vi "manip_linearize.vi"(6 "Reset":bool, 7 "Parameters":T1={"Stimulus"={"Type"=enum."Off", "Phase"=0.0, "Amplitude"=[], "Injection point"=enum."Total pose", "Closed loop"=FALSE, "Offset"=[], "Tip -> world"=FALSE, "Frequency"=0.0, "Length"=0.0}, "Goal Filter A"={"Speedup max"=0.0, "Speedup thresh"=0.0, "Speedup nonlin"=0.0, "Filters"=[]}, "Mode controls"={"Hold"=FALSE, "Cancellation"=FALSE, "Goal filter"=FALSE, "Trigger"=FALSE}, "Manipulator type"=enum."Current piezo", "Manipulator calibration"={"Tool offsets"=[[0.0, 0.0, 36200.0]], "Tip light calibration"=[], "Handle light calibration"=[], "Base pivots"=[], "Output pivots"=[], "Length center"=0.0, "Workspace height"=[], "Workspace diameter"=[0.0, 0.0, 36200.0], "Linearization"=[[0.0, 0.0, 36200.0]], "Stack travel"=400.0, "Saturation pos"=375.0, "Inverse filters"=[]}, "Network"={"Remote Host"="", "Send Status"=FALSE, "Send Port"=0, "Recv Commands"=FALSE, "Recv Port"=0}, "Goal Filter B"={"Speedup max"=0.0, "Speedup thresh"=0.0, "Speedup nonlin"=0.0, "Filters"=[]}, "Cancellation"={"KP"={"XY"=0.0, "Rxy"=0.0, "Z"=0.0, "Rz"=0.0}, "KI"=0.0, "KD"={"XY"=0.0, "Rxy"=0.0, "Z"=0.0, "Rz"=0.0}, "Max vel"=20.0, "Max acc"=0.001, "Int error limit"=3.0, "RCM gain"=0.0, "Bypass"=FALSE, "Degraded gain"=0.0}, "Transition time"=0.0, "Estimation"={"Link"={"Measure noise"=[], "Process noise"=[], "Alt process noise"=[], "Alt turnoff cycles"=20, "Innovation limit"=[], "Residue threshold"=0.0, "Enable"=FALSE}, "Handle"={"Measure noise"=[], "Process noise"=[], "State limits"=[], "Innovation limit"=[], "Prediction Lookahead"=0.0, "Enable"=FALSE}}} {"Transition time" format="%_3f"; "Cancellation"."Degraded gain" min=0 max=1 step=0.1 format="%#_3p"; "Cancellation"."RCM gain" min=0 max=1 step=0.1 format="%#_3p"; "Cancellation"."KD"."Rz" min=0 max=1 step=0.1 format="%#_3p"; "Cancellation"."KD"."Rxy" min=0 max=1 step=0.1 format="%#_3p"; "Cancellation"."KD"."Z" min=0 max=1 step=0.1 format="%#_3p"; "Cancellation"."KD"."XY" min=0 max=1 step=0.1 format="%#_3p"; "Cancellation"."KI" min=0 max=1 step=0.01 format="%#_3p"; "Cancellation"."KP"."Rz" min=0 max=1 step=0.1 format="%#_3p"; "Cancellation"."KP"."Rxy" min=0 max=1 step=0.1 format="%#_3p"; "Cancellation"."KP"."Z" min=0 max=1 step=0.1 format="%#_3p"; "Cancellation"."KP"."XY" min=0 max=1 step=0.1 format="%#_3p"; "Cancellation"."Max acc" format="%#_3p"; "Goal Filter B"."Filters"."V limit range" format="%_3p"; "Goal Filter B"."Filters"."V limit" format="%_3p"; "Goal Filter B"."Filters"."Upper Q" format="%_3f"; "Goal Filter B"."Filters"."Upper Fc" format="%_3p"; "Goal Filter B"."Filters"."Lower Q" format="%_3f"; "Goal Filter B"."Filters"."Scale factor" format="%_3f"; "Goal Filter B"."Filters"."Lower Fc" format="%_3p"; "Goal Filter B"."Speedup nonlin" format="%_3p"; "Goal Filter B"."Speedup thresh" format="%_3p"; "Goal Filter B"."Speedup max" format="%_3p"; "Manipulator calibration"."Saturation pos" format="%#.1f"; "Manipulator calibration"."Stack travel" format="%#.1f"; "Manipulator calibration"."Output pivots" format="%#_6f"; "Manipulator calibration"."Base pivots" format="%#_6f"; "Manipulator calibration"."Handle light calibration" format="%#.1f"; "Manipulator calibration"."Tip light calibration" format="%#.1f"; "Goal Filter A"."Filters"."V limit range" format="%_3p"; "Goal Filter A"."Filters"."V limit" format="%_3p"; "Goal Filter A"."Filters"."Upper Q" format="%_3f"; "Goal Filter A"."Filters"."Upper Fc" format="%_3p"; "Goal Filter A"."Filters"."Lower Q" format="%_3f"; "Goal Filter A"."Filters"."Scale factor" format="%_3f"; "Goal Filter A"."Filters"."Lower Fc" format="%_3p"; "Goal Filter A"."Speedup nonlin" format="%_3p"; "Goal Filter A"."Speedup thresh" format="%_3p"; "Goal Filter A"."Speedup max" format="%_3p"; "Stimulus"."Length" min=0.0 max=100.0 step=100.0 format="%#_4p"; "Stimulus"."Frequency" min=0.0 step=100.0 format="%#_4g"; "Stimulus"."Offset" format="%#_3p"; "Stimulus"."Amplitude" format="%#_3p"; "Stimulus"."Phase" min=-180.0 max=360.0 step=100.0 format="%#.2f"}, 9 "Input":sgl[](array[numeric])) -> (0 "Saturation":bool[](array[boolean]), 1 "Output":sgl[](array[numeric]))   [LabVIEW 2013]
uses:
  testing/Micron params.ctl
  testing/stimulus.ctl
  testing/injection_point.ctl
  filtering/goal_loop_parms.ctl
  testing/mode_conrols.ctl
  testing/manipulator_cal.ctl
  asap/labview/testing/probe_calibration.ctl
  host/network_params.ctl
  sq_control_params.ctl
  decoupled_gain.ctl
  estimation_controls.ctl
  <vilib>/Analysis/1siggen.llb/Ramp Pattern by Samples.vi
  <vilib>/Analysis/polynomials.llb/1D Polynomial Evaluation (DBL).vi
  <vilib>/Analysis/NI_AALBase.lvlib
  <vilib>/Analysis/NI_AALPro.lvlib
  <vilib>/gmath/NI_Gmath.lvlib
panel:
  in  "Enable":bool=TRUE
  out "X":dbl[][](array[numeric])
  out "Y":dbl[](array[numeric])
  in  "Linearization":sgl[][](array[numeric])
  # "Locals:"
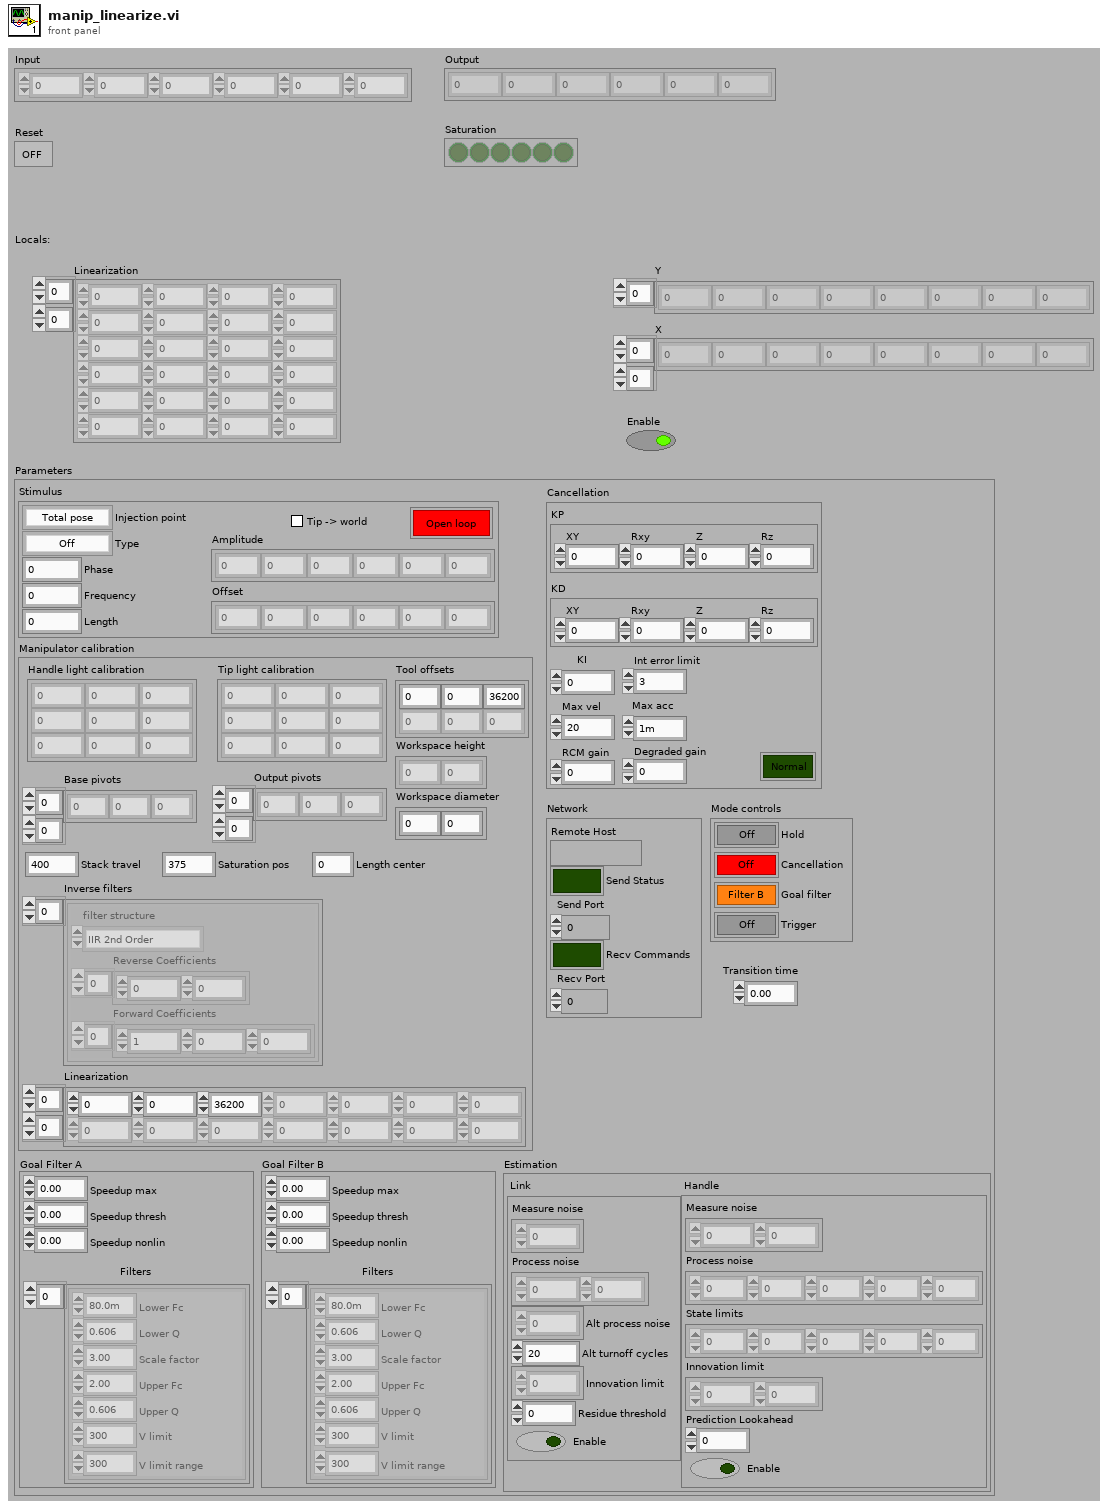
[diagram p1: front panel]
types:
  T1 = typedef "Micron params.ctl" = cluster{"Stimulus":T2, "Goal Filter A":T4, "Mode controls":T5, "Manipulator type":enum16{"Current piezo", "Voltage piezo"}, "Manipulator calibration":T6, "Network":T8, "Goal Filter B":T4, "Cancellation":T9, "Transition time":sgl, "Estimation":T11}
  T2 = typedef "stimulus.ctl" = cluster{"Type":enum16{"Off", "Step", "Sine", "Triangle", "Arbitrary"}, "Phase":dbl, "Amplitude":sgl[], "Injection point":T3, "Closed loop":bool, "Offset":sgl[], "Tip -> world":bool, "Frequency":dbl, "Length":dbl}
  T3 = typedef "injection_point.ctl" = enum16{"Total pose", "V limiter", "Goal ", "Link position", "KF link position", "Inverse kin", "Link goal", "Link error", "Controller", "Output", "Drive", "Light"}
  T4 = typedef "goal_loop_parms.ctl" = cluster{"Speedup max":sgl, "Speedup thresh":sgl, "Speedup nonlin":sgl, "Filters":cluster{"Lower Fc":sgl, "Lower Q":sgl, "Scale factor":sgl, "Upper Fc":sgl, "Upper Q":sgl, "V limit":sgl, "V limit range":sgl}[]}
  T5 = typedef "mode_conrols.ctl" = cluster{"Hold":bool, "Cancellation":bool, "Goal filter":bool, "Trigger":bool}
  T6 = typedef "manipulator_cal.ctl" = cluster{"Tool offsets":sgl[][], "Tip light calibration":T7, "Handle light calibration":T7, "Base pivots":sgl[][], "Output pivots":sgl[][], "Length center":sgl, "Workspace height":sgl[], "Workspace diameter":sgl[], "Linearization":sgl[][], "Stack travel":sgl, "Saturation pos":sgl, "Inverse filters":cluster{"filter structure":enum32{"IIR 2nd Order", "IIR 4th Order"}, "Reverse Coefficients":dbl[], "Forward Coefficients":dbl[]}[]}
  T7 = typedef "probe_calibration.ctl" = sgl[][]
  T8 = typedef "network_params.ctl" = cluster{"Remote Host":string, "Send Status":bool, "Send Port":u16, "Recv Commands":bool, "Recv Port":u16}
  T9 = typedef "sq_control_params.ctl" = cluster{"KP":T10, "KI":sgl, "KD":T10, "Max vel":sgl, "Max acc":sgl, "Int error limit":sgl, "RCM gain":sgl, "Bypass":bool, "Degraded gain":sgl}
  T10 = typedef "decoupled_gain.ctl" = cluster{"XY":sgl, "Rxy":sgl, "Z":sgl, "Rz":sgl}
  T11 = typedef "estimation_controls.ctl" = cluster{"Link":cluster{"Measure noise":dbl[], "Process noise":dbl[], "Alt process noise":dbl[], "Alt turnoff cycles":i32, "Innovation limit":dbl[], "Residue threshold":dbl, "Enable":bool}, "Handle":cluster{"Measure noise":dbl[], "Process noise":dbl[], "State limits":dbl[], "Innovation limit":dbl[], "Prediction Lookahead":sgl, "Enable":bool}}
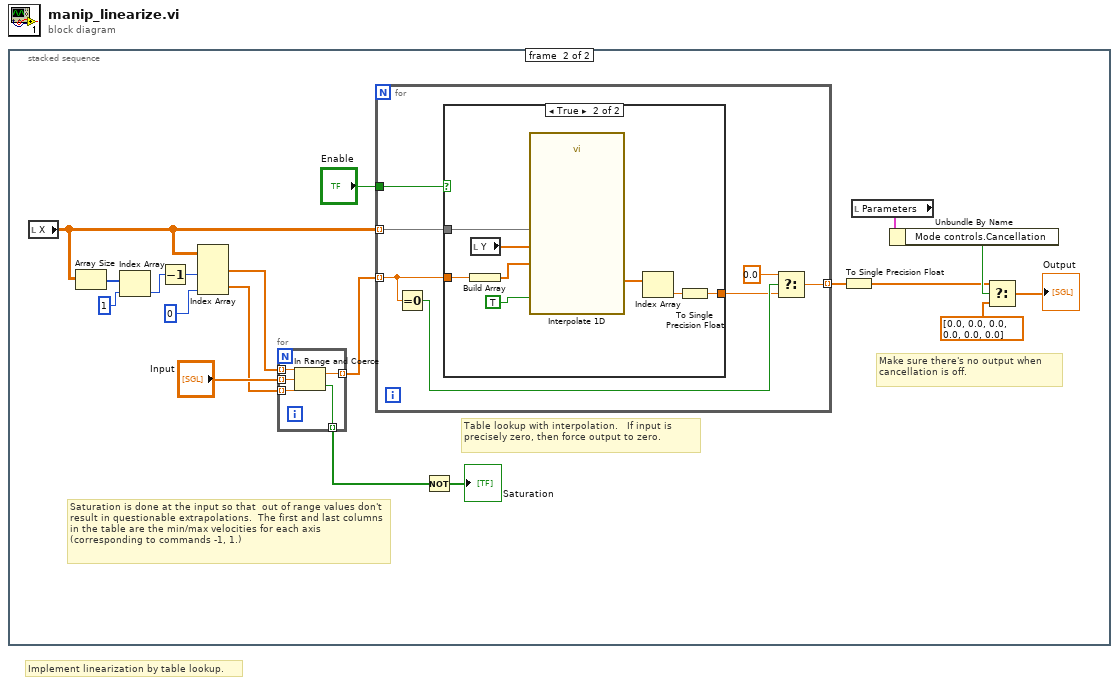
[diagram p0: block diagram]
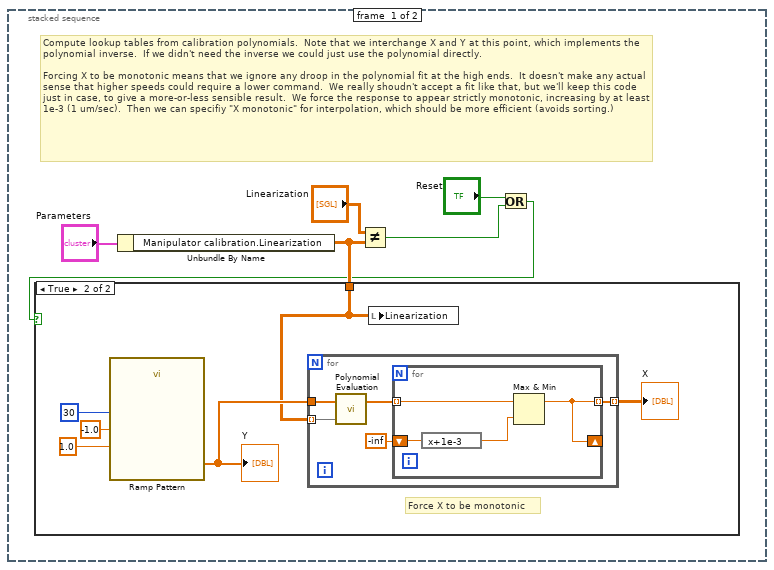
[diagram p2: hidden frame]
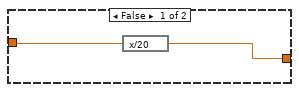
[diagram p4: hidden frame]
diagram:
  # "Implement linearization by table lookup."
  n1 = stacked-sequence {
    frame #0 {
      # "Compute lookup tables from calibration polynomials.  Note that we interchange X and Y at this point, which implements the polynomial inverse.  If we didn't need the inverse we could just use the polynomial directly.\n\nForcing X to be monotonic means that we ignore any droop in the polynomial fit at the high ends.  It doesn't make any actual sense that higher speeds could require a lower command.  We really shoudn't accept a fit like that, but we'll keep this code just in case, to give a more-or-less sensible result.  We force the response to appear strictly monotonic, increasing by at least 1e-3 (1 um/sec).  Then we can specifiy \"X monotonic\" for interpolation, which should be more efficient (avoids sorting.)"
      n2 = Unbundle By Name("Parameters") -> ("Manipulator calibration.Linearization"=w4:sgl[][])
      n3 = Not Equal?(x="Linearization", y=w4) -> (x != y?=w2:bool)
      n4 = Or(x="Reset", y=w2) -> (x .or. y?=w1:bool)
      n5 = case shown="True" w1 {
        tunnel: w4 -> [_ w8]
        frame False {
        }
        frame True {
          # "Force X to be monotonic"
          n6 = call-poly <vilib>:"Ramp Pattern.vi"("start"=-1.0, "end"=1.0, "samples"=30) -> ("Ramp Pattern"=w9:dbl[])  [unwired: 7 in, 1 out]
          "Y" <- w9
          n7 = for {
            tunnel: w9 -> [w17]
            tunnel: w8 -> [w16] mode=indexing
            tunnel: [w13] -> w7 mode=indexing
            n8 = call-poly <vilib>:"Polynomial Evaluation.vi"("P(x)"=w16, "A"=w17) -> ("P(A)"=w15:dbl[])  [unwired: 1 out]
            n9 = for {
              tunnel: w15 -> [w21] mode=indexing
              shift-right: [w20] -> _
              shift-left: -inf -> [w19]
              tunnel: [w20] -> w13 mode=indexing
              n10 = expression code="x+1e-3"(w19) -> (w18:dbl)
              n11 = Max & Min(x=w21, y=w18) -> (max(x,y)=w20:dbl)  [unwired: 1 out]
            }
          }
          "X" <- w7
          n12 = local write "Linearization"(w8) -> ()
        }
      }
    }
    frame #1 {
      # "Saturation is done at the input so that  out of range values don't result in questionable extrapolations.  The first and last columns in the table are the min/max velocities for each axis (corresponding to commands -1, 1.)"
      # "Table lookup with interpolation.   If input is  precisely zero, then force output to zero."
      # "Make sure there's no output when cancellation is off."
      n13 = local read "X"() -> (w31:dbl[][])
      n14 = Array Size(array=w31) -> (size(s)=w32:i32[])
      n15 = Index Array(array=w32, index=1) -> (element=w23:i32)
      n16 = Decrement(x=w23) -> (x-1=w22:i32)
      n17 = Index Array(array=w31, index (col) #1=w22, index (col) #2=0 ("index (col)")) -> (element #1=w30:dbl[], element #2=w29:dbl[])  [unwired: 2 in]
      n18 = for {
        tunnel: [w45] -> w35 mode=indexing
        tunnel: "Input" -> [w44] mode=indexing
        tunnel: w30 -> [w43] mode=indexing
        tunnel: w29 -> [w42] mode=indexing
        tunnel: [w41] -> w28 mode=indexing
        n19 = In Range and Coerce(upper limit=w43, x=w44, lower limit=w42) -> (coerced(x)=w41:dbl, In Range?=w45:bool)
      }
      n20 = for {
        tunnel: w31 -> [w52] mode=indexing
        tunnel: w28 -> [w50] mode=indexing
        tunnel: [w46] -> w25 mode=indexing
        tunnel: "Enable" -> [w51]
        n21 = Equal To 0?(x=w50) -> (x = 0?=w49:bool)
        n22 = case shown="True" w51 {
          tunnel: w52 -> [_ w62]
          tunnel: w50 -> [w54 w61]
          tunnel: [w53 w55] -> w47
          frame False {
            n23 = expression code="x/20"(w54) -> (w53:dbl)
          }
          frame True {
            n24 = Build Array(w61) -> (w59:dbl[])
            n25 = local read "Y"() -> (w60:dbl[])
            n26 = call <vilib>:"Interpolate 1D.vi"("X is monotonic"=TRUE, "xi"=w59, "X"=w62, "Y"=w60) -> ("yi"=w57:dbl[])  [unwired: 5 in, 2 out]
            n27 = Index Array(array=w57) -> (element=w56:dbl)  [unwired: 1 in]
            n28 = To Single Precision Float(number=w56) -> (single precision float=w55:sgl)
          }
        }
        n29 = Select(t=0.0, s=w49, f=w47) -> (s? t:f=w46:dbl)
      }
      n30 = Not(x=w35) -> (.not. x?=→"Saturation":bool[])
      n31 = To Single Precision Float(number=w25) -> (single precision float=w26:sgl[])
      n32 = local read "Parameters"() -> (w38:T1)
      n33 = Unbundle By Name(w38) -> ("Mode controls.Cancellation"=w37:bool)
      n34 = Select(t=w26, s=w37, f=sgl[] [0.0, 0.0, 0.0, 0.0, 0.0, 0.0]) -> (s? t:f=→"Output":sgl[])
    }
  }
